vi "solar_voy_def Import (Empty).vi"(5 "Endian (BIG)":enum8{"BIG", "LITTLE"}(ring), 6 "Suppress Errors? (T)":bool=TRUE, 8 "error in (no error)":errorcluster, 9 "TLM Packet Names":string[](array[string]), 10 "CMD Packet Names":string[](array[string]), 11 "Target Name":string) -> (0 "error out":errorcluster, 3 "PACKETS":T1[](array[typedef]) {"last_time" format="%<%H:%M:%S%3u %m/%d/%y>T"})   [LabVIEW 2018]
doc: "This imports empty command and telemetry packets and includes a 'DUMMY' parameter/item required by COSMOS.\n\nTo add a description, add \",d=Description here\" to the packet name."
uses:
  solar_voy_def_ctl ITEM TYPE.ctl
  type/solar_type Item Type.ctl
  solar_voy_def_ctl ITEM (Simple).ctl
  solar_voy_def_ctl ITEM.ctl
  solar_voy_def_ctl PACKET_ID.ctl
  solar_voy_def_ctl PACKET.ctl
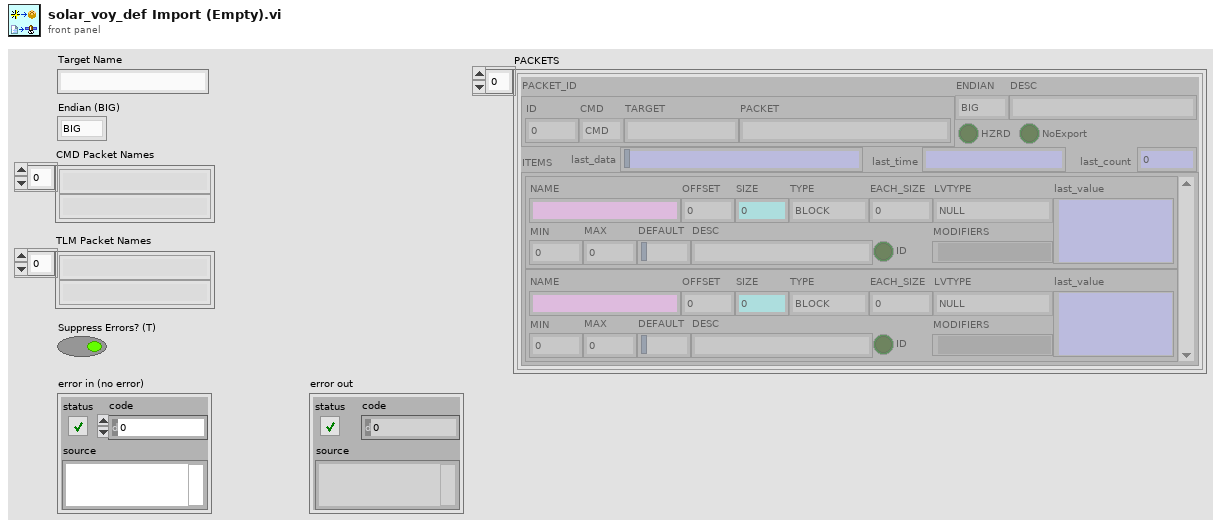
[diagram p1: front panel]
types:
  T1 = typedef "solar_voy_def_ctl PACKET.ctl" = cluster{"PACKET_ID":T2, "ENDIAN":enum8{"BIG", "LITTLE"}, "DESC":string, "HZRD":bool, "ITEMS":T3[], "NoExport":bool, "last_time":timestamp, "last_count":u32, "last_data":string}
  T2 = typedef "solar_voy_def_ctl PACKET_ID.ctl" = cluster{"ID":u16, "CMD":enum8{"CMD", "TLM"}, "TARGET":string, "PACKET":string}
  T3 = typedef "solar_voy_def_ctl ITEM.ctl" = cluster{"NAME":string, "OFFSET":i32, "SIZE":i32, "TYPE":T4, "EACH_SIZE":i32, "LVTYPE":T5, "MIN":dbl, "MAX":dbl, "DEFAULT":string, "DESC":string, "ID":bool, "MODIFIERS":variant, "last_value":variant}
  T4 = typedef "solar_voy_def_ctl ITEM TYPE.ctl" = enum8{"BLOCK", "INT", "UINT", "FLOAT", "STRING"}
  T5 = typedef "solar_type Item Type.ctl" = enum16{"NULL", "UNKNOWN", "CLUSTER", "I8", "I16", "I32", "I64", "U8", "U16", "U32", "U64", "U8_ENUM", "U16_ENUM", "U32_ENUM", "SGL", "DBL", "BOOLEAN", "STRING", "PATH", "VISA", "TAG", "TIME", "I8_1D", "I16_1D", "I32_1D", "I64_1D", "U8_1D", "U16_1D", "U32_1D", "U64_1D", "U8_ENUM_1D", "U16_ENUM_1D", "U32_ENUM_1D", "SGL_1D", "DBL_1D", "BOOLEAN_1D", "STRING_1D", "PATH_1D", "VISA_1D", "TAG_1D", "TIME_1D", "I8_2D", "I16_2D", "I32_2D", "I64_2D", "U8_2D", "U16_2D", "U32_2D", "U64_2D", "U8_ENUM_2D", "U16_ENUM_2D", "U32_ENUM_2D", "SGL_2D", "DBL_2D", "BOOLEAN_2D", "STRING_2D", "PATH_2D", "VISA_2D", "TAG_2D", "TIME_2D"}
  T6 = typedef "solar_voy_def_ctl ITEM (Simple).ctl" = cluster{"NAME":string, "LVTYPE":T5, "BIT_SIZE":i32, "TYPE":T4, "DEFAULT":string, "EACH_SIZE":i32, "ID":bool, "STATES(k,v)":string[][], "DESC":string}
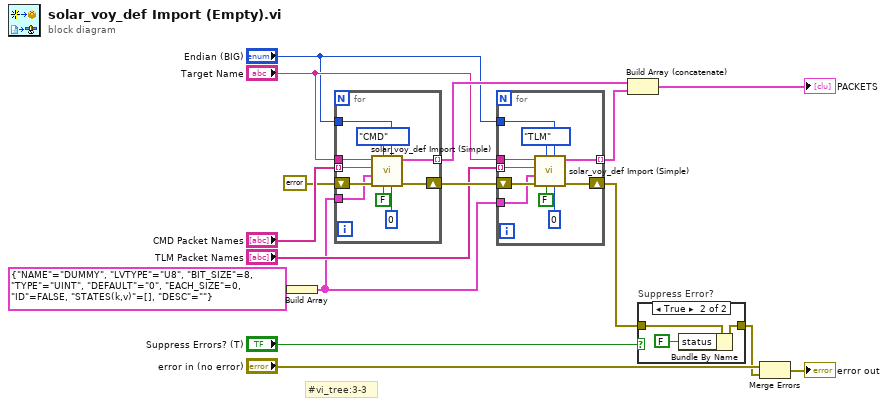
[diagram p0: block diagram]
diagram:
  # "#vi_tree:3-3"
  n1 = Build Array(T6 {"NAME"="DUMMY", "LVTYPE"=enum."U8", "BIT_SIZE"=8, "TYPE"=enum."UINT", "DEFAULT"="0", "EACH_SIZE"=0, "ID"=FALSE, "STATES(k,v)"=[], "DESC"=""} ("ITEM (Simple)")) -> (w1:T6[])
  n2 = for {
    tunnel: "Target Name" -> [w25]
    shift-right: [w22] -> w14
    shift-left: errorcluster {"status"=FALSE, "code"=0, "source"=""} ("error out") -> [w26]
    tunnel: "CMD Packet Names" -> [w18] mode=indexing
    tunnel: "Endian (BIG)" -> [w23]
    tunnel: [w21] -> w15 mode=indexing
    tunnel: w1 -> [w17]
    n3 = call "solar_voy_def Import (Simple).vi"("Default ID"=u16 0 ("Default ID (0=Create)"), "Endian (BIG)"=w23, "Suppress Errors? (T)"=FALSE, "CMD"=enum8{"CMD", "TLM"}."CMD", "error in (no error)"=w26, "ITEMS (Simple)"=w17, "PACKET"=w18, "TARGET"=w25) -> ("error out"=w22:errorcluster, "PACKET"=w21:T1)  [unwired: 2 in]
  }
  n4 = for {
    tunnel: "Target Name" -> [w35]
    shift-right: [w31] -> w6
    shift-left: w14 -> [w36]
    tunnel: "TLM Packet Names" -> [w34] mode=indexing
    tunnel: "Endian (BIG)" -> [w32]
    tunnel: [w30] -> w11 mode=indexing
    tunnel: w1 -> [w27]
    n5 = call "solar_voy_def Import (Simple).vi"("Default ID"=u16 0 ("Default ID (0=Create)"), "Endian (BIG)"=w32, "Suppress Errors? (T)"=FALSE, "CMD"=enum8{"CMD", "TLM"}."TLM", "error in (no error)"=w36, "ITEMS (Simple)"=w27, "PACKET"=w34, "TARGET"=w35) -> ("error out"=w31:errorcluster, "PACKET"=w30:T1)  [unwired: 2 in]
  }
  n6 = Build Array (concatenate)(w15, w11) -> (→"PACKETS":T1[])
  n7 = case "Suppress Error?" shown="True" "Suppress Errors? (T)" {
    tunnel: w6 -> [w37 w40]
    tunnel: [w37 w39] -> w4
    frame False {
    }
    frame True {
      n8 = Bundle By Name(cluster=w40, "status"=FALSE) -> (w39:errorcluster)
    }
  }
  n9 = Merge Errors("error in (no error)", w4) -> (→"error out":errorcluster)
